vi "Plot Zoom Key Down Detect.vi"(8 "error in (no error)":errorcluster, 10 "Refs":T12, 11 "Loop data in":T1={"TitleCollapse"=refnum, "MouseDownState"=enum."Idle", "RightClickCache"={"Mod"={"Ctrl"=FALSE, "Shift"=FALSE}, "CoordsStart"={"Horizontal"=0, "Vertical"=0}, "CoordsEnd"={"Horizontal"=0, "Vertical"=0}, "PlotAreaBounds"={"Left"=10, "Top"=10, "Right"=0, "Bottom"=0}, "slice"=[]}, "ZoomCache"={"SuppressedPlots"=[], "LeftAxis"={"NeedsRevert?"=FALSE, "Scale Fit"=0, "Range"={"Minimum"=0.0, "Maximum"=0.0, "Increment"=0.0, "Minor Increment"=0.0, "Start"=0.0}}, "RightAxis"={"NeedsRevert?"=FALSE, "Scale Fit"=0, "Range"={"Minimum"=0.0, "Maximum"=0.0, "Increment"=0.0, "Minor Increment"=0.0, "Start"=0.0}}, "Mod"={"Shift"=FALSE}}, "UpdateTime"=0.0, "keyboard"=refnum, "visible?"=FALSE}) -> (0 "error out":errorcluster, 3 "Loop data out":T1={"TitleCollapse"=refnum, "MouseDownState"=enum."Idle", "RightClickCache"={"Mod"={"Ctrl"=FALSE, "Shift"=FALSE}, "CoordsStart"={"Horizontal"=0, "Vertical"=0}, "CoordsEnd"={"Horizontal"=0, "Vertical"=0}, "PlotAreaBounds"={"Left"=10, "Top"=10, "Right"=0, "Bottom"=0}, "slice"=[]}, "ZoomCache"={"SuppressedPlots"=[], "LeftAxis"={"NeedsRevert?"=FALSE, "Scale Fit"=0, "Range"={"Minimum"=0.0, "Maximum"=0.0, "Increment"=0.0, "Minor Increment"=0.0, "Start"=0.0}}, "RightAxis"={"NeedsRevert?"=FALSE, "Scale Fit"=0, "Range"={"Minimum"=0.0, "Maximum"=0.0, "Increment"=0.0, "Minor Increment"=0.0, "Start"=0.0}}, "Mod"={"Shift"=FALSE}}, "UpdateTime"=0.0, "keyboard"=refnum, "visible?"=FALSE})   [LabVIEW 2021, in "RocketPlot.lvlib"]
uses:
  RocketPlot.lvlib
  TypeDefs/Plot UI references.ctl
  Classes/RocketPlotHandle/RocketPlotHandle.lvclass
  <userlib>/bjustice/TipStripOOPanel/Classes/TipPanelHandle/TipPanelHandle.lvclass
  TypeDefs/Plot top row.ctl
  TypeDefs/plot while loop data.ctl
  CollapsePanel/CollapsePanel.lvclass
  TypeDefs/MouseDownState.ctl
  TypeDefs/RightClickCache.ctl
  TypeDefs/RightClickCache PlatMod.ctl
  <vilib>/Utility/miscctls.llb/LVPoint32TypeDef.ctl
  <vilib>/Utility/miscctls.llb/LVRectTypeDef.ctl
  TypeDefs/Slice average.ctl
  TypeDefs/ZoomCache.ctl
  TypeDefs/RangeCache.ctl
  <vilib>/Utility/miscctls.llb/LVRangeTypeDef.ctl
  TypeDefs/ZoomCache PlatMod.ctl
  PlatMods to Zoom mods.vi
  <vilib>/Utility/inputDevices.llb/keyboardAcquire.vi
  Zoom Cache end.vi
  Zoom Cache start.vi
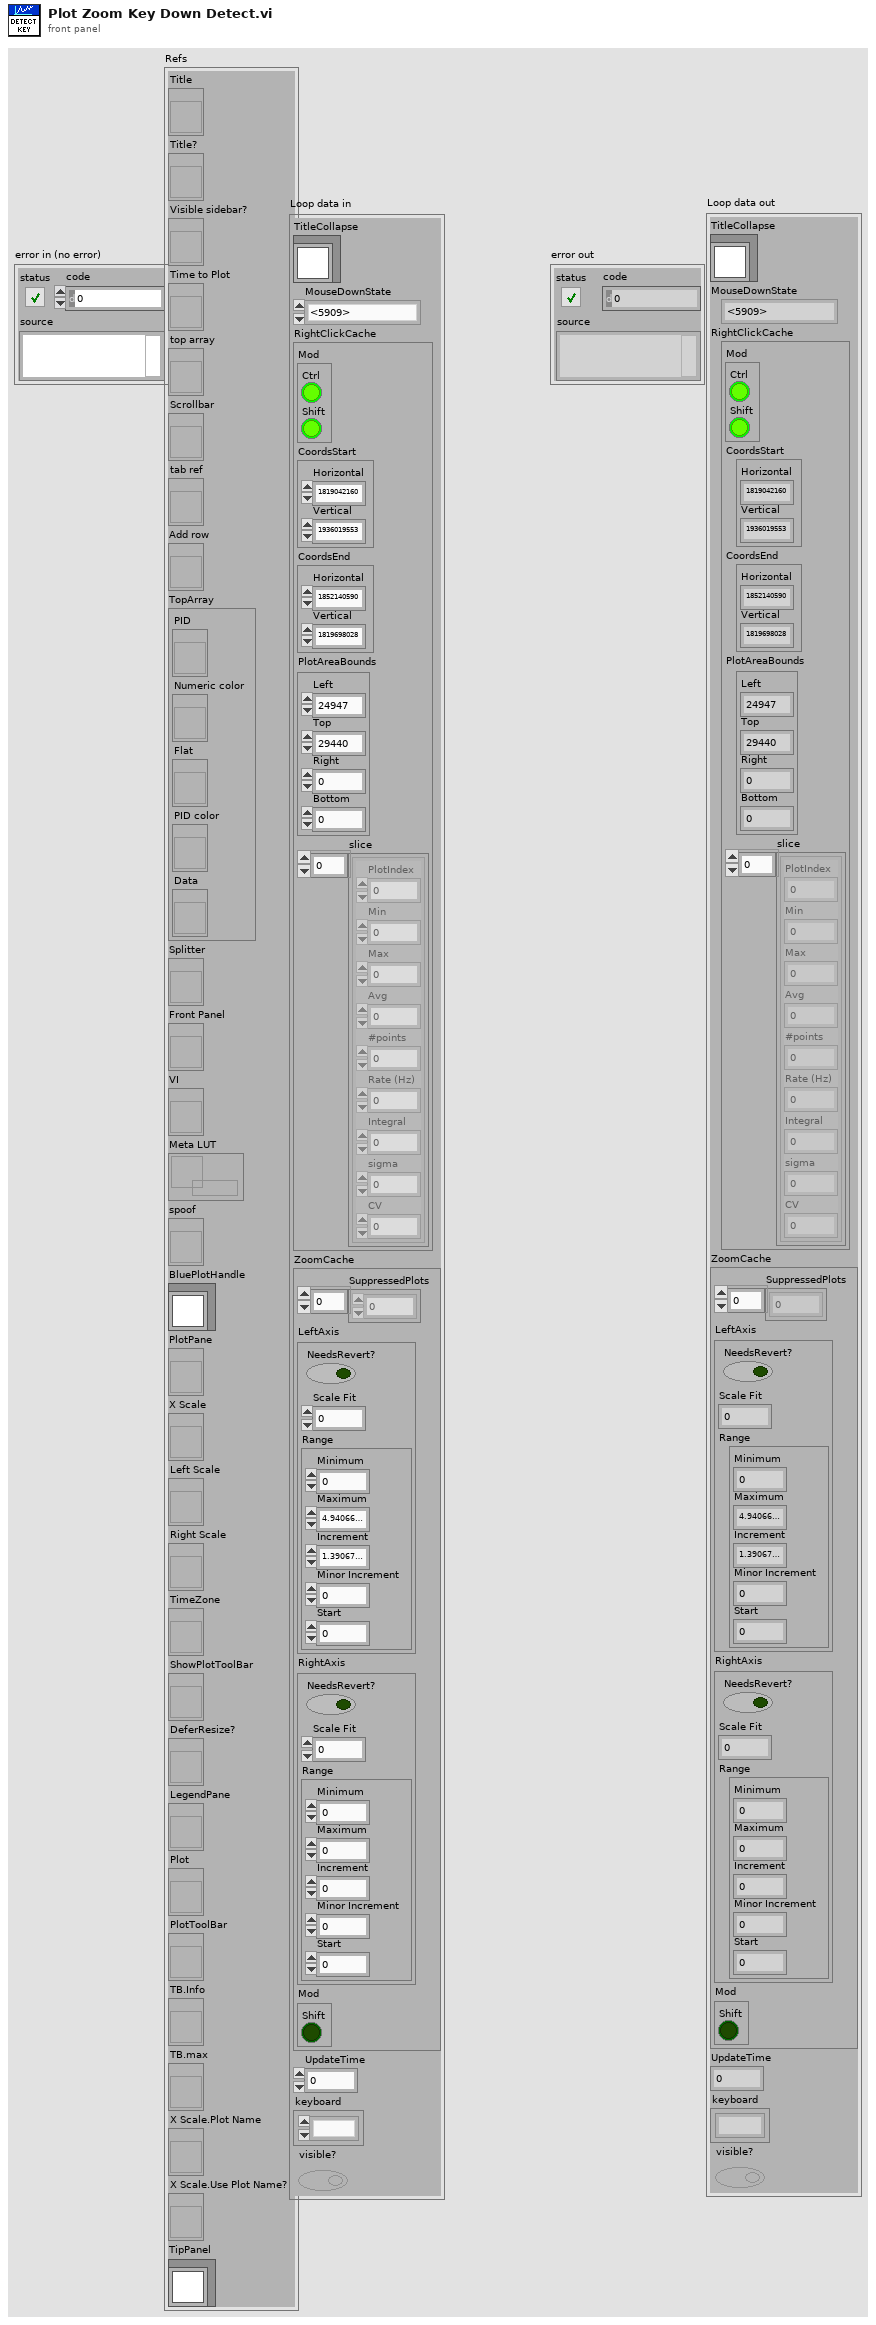
[diagram p1: front panel]
types:
  T1 = typedef "RocketPlot.lvlib/plot while loop data.ctl" = cluster{"TitleCollapse":refnum<class "CollapsePanel.lvclass">, "MouseDownState":T2, "RightClickCache":T3, "ZoomCache":T8, "UpdateTime":dbl, "keyboard":refnum<k1>, "visible?":bool}
  T2 = typedef "RocketPlot.lvlib/MouseDownState.ctl" = enum16{"Idle", "Pan", "Zoom", "Zoom-Post", "RightClick"}
  T3 = typedef "RocketPlot.lvlib/RightClickCache.ctl" = cluster{"Mod":T4, "CoordsStart":T5, "CoordsEnd":T5, "PlotAreaBounds":T6, "slice":T7[]}
  T4 = typedef "RocketPlot.lvlib/RightClickCache PlatMod.ctl" = cluster{"Ctrl":bool, "Shift":bool}
  T5 = typedef "LVPoint32TypeDef.ctl" = cluster{"Horizontal":i32, "Vertical":i32}
  T6 = typedef "LVRectTypeDef.ctl" = cluster{"Left":i16, "Top":i16, "Right":i16, "Bottom":i16}
  T7 = typedef "RocketPlot.lvlib/Slice average.ctl" = cluster{"PlotIndex":i32, "Min":dbl, "Max":dbl, "Avg":dbl, "#points":u32, "Rate (Hz)":dbl, "Integral":dbl, "sigma":dbl, "CV":dbl}
  T8 = typedef "RocketPlot.lvlib/ZoomCache.ctl" = cluster{"SuppressedPlots":i32[], "LeftAxis":T9, "RightAxis":T9, "Mod":T11}
  T9 = typedef "RocketPlot.lvlib/RangeCache.ctl" = cluster{"NeedsRevert?":bool, "Scale Fit":u8, "Range":T10}
  T10 = typedef "LVRangeTypeDef.ctl" = cluster{"Minimum":dbl, "Maximum":dbl, "Increment":dbl, "Minor Increment":dbl, "Start":dbl}
  T11 = typedef "RocketPlot.lvlib/ZoomCache PlatMod.ctl" = cluster{"Shift":bool}
  T12 = typedef "RocketPlot.lvlib/Plot UI references.ctl" = cluster{"Title":refnum<vi>, "Title?":refnum<vi>, "Visible sidebar?":refnum<vi>, "Time to Plot":refnum<vi>, "top array":refnum<vi>, "Scrollbar":refnum<vi>, "tab ref":refnum<vi>, "Add row":refnum<vi>, "TopArray":cluster{"PID":refnum<vi>, "Numeric color":refnum<vi>, "Flat":refnum<vi>, "PID color":refnum<vi>, "Data":refnum<vi>}, "Splitter":refnum<vi>, "Front Panel":refnum<vi>, "VI":refnum<vi>, "Meta LUT":refnum<data-value>, "spoof":refnum<vi>, "BluePlotHandle":refnum<class "RocketPlotHandle.lvclass">, "PlotPane":refnum<vi>, "X Scale":refnum<vi>, "Left Scale":refnum<vi>, "Right Scale":refnum<vi>, "TimeZone":refnum<vi>, "ShowPlotToolBar":refnum<vi>, "DeferResize?":refnum<vi>, "LegendPane":refnum<vi>, "Plot":refnum<vi>, "PlotToolBar":refnum<vi>, "TB.Info":refnum<vi>, "TB.max":refnum<vi>, "X Scale.Plot Name":refnum<vi>, "X Scale.Use Plot Name?":refnum<vi>, "TipPanel":refnum<class "TipPanelHandle.lvclass">}
  T13 = cluster{"Shift":bool, "Ctrl":bool, "Alt":bool, "Cmd":bool, "Opt":bool}
  T14 = enum16{"0", "1", "2", "3", "4", "5", "6", "7", "8", "9", "A", "B", "C", "D", "E", "F", "G", "H", "I", "J", "K", "L", "M", "N", "O", "P", "Q", "R", "S", "T", "U", "V", "W", "X", "Y", "Z", "F1", "F2", "F3", "F4", "F5", "F6", "F7", "F8", "F9", "F10", "F11", "F12", "F13", "F14", "F15", "ADD", "BACK", "BACKSLASH", "CAPITAL", "COMMA", "DECIMAL", "DELETE", "DIVIDE", "DOWN", "END", "EQUALS", "ESCAPE", "GRAVE (`)", "HOME", "INSERT", "LBRACKET", "LCONTROL", "LEFT", "L ALT", "LSHIFT", "LWIN", "MINUS", "MULTIPLY", "NEXT", "NUMLOCK", "NUMPAD_0", "NUMPAD_1", "NUMPAD_2", "NUMPAD_3", "NUMPAD_4", "NUMPAD_5", "NUMPAD_6", "NUMPAD_7", "NUMPAD_8", "NUMPAD_9", "PAUSE", "PERIOD", "PRIOR (PG UP)", "RBRACKET", "RCONTROL", "RETURN", "RIGHT", "R ALT", "RSHIFT", "RWIN", "SCROLL", "SEMICOLON", "SLASH", "SPACE", "SUBTRACT", "TAB", "UP", "ENTER (num pad)", "' (quote)"}
  T15 = enum16{"0", "1", "2", "3", "4", "5", "6", "7", "8", "9", "A", "B", "C", "D", "E", "F", "G", "H", "I", "J", "K", "L", "M", "N", "O", "P", "Q", "R", "S", "T", "U", "V", "W", "X", "Y", "Z", "F1", "F2", "F3", "F4", "F5", "F6", "F7", "F8", "F9", "F10", "F11", "F12", "F13", "F14", "F15", "ADD", "BACK", "BACKSLASH", "CAPITAL", "COMMA", "DECIMAL", "DELETE", "DIVIDE", "DOWN", "END", "EQUALS", "ESCAPE", "GRAVE (`)", "HOME", "INSERT", "LBRACKET", "LCONTROL", "LEFT", "L ALT", "LSHIFT", "LWIN", "MINUS", "MULTIPLY", "NEXT", "NUMLOCK", "NUMPAD_0", "NUMPAD_1", "NUMPAD_2", "NUMPAD_3", "NUMPAD_4", "NUMPAD_5", "NUMPAD_6", "NUMPAD_7", "NUMPAD_8", "NUMPAD_9", "PAUSE", "PERIOD", "PRIOR (PG UP)", "RBRACKET", "RCONTROL", "RETURN", "RIGHT", "R ALT", "RSHIFT", "RWIN", "SCROLL", "SEMICOLON", "SLASH", "SPACE", "SUBTRACT", "TAB", "UP", "ENTER (num pad)", "' (quote)"}[]
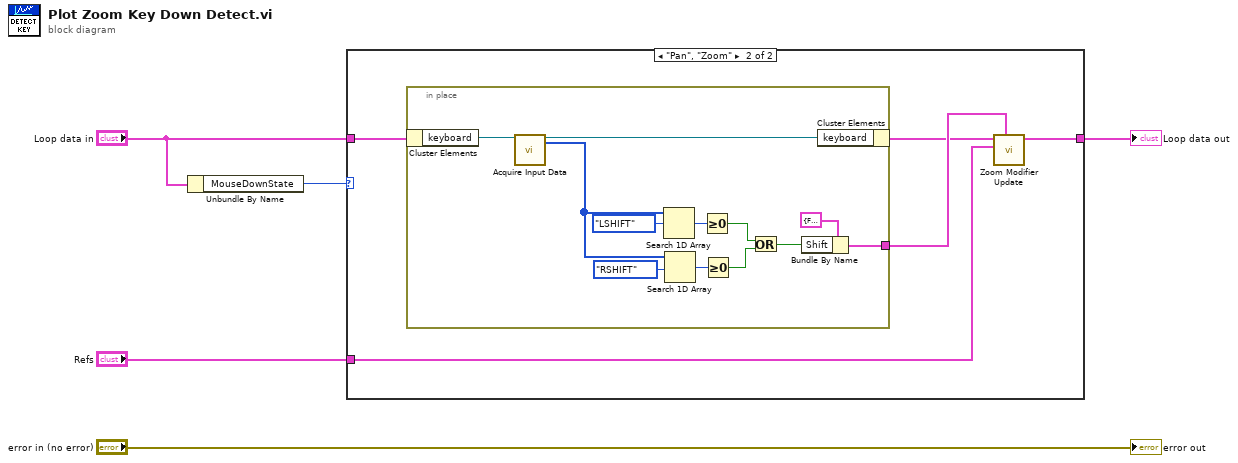
[diagram p0: block diagram]
diagram:
  n1 = Unbundle By Name("Loop data in") -> ("MouseDownState"=w1:T2)
  n2 = case shown="\"Pan\", \"Zoom\"" w1 {
    tunnel: [w6 w9] -> w4
    tunnel: "Refs" -> [_ w11]
    tunnel: "Loop data in" -> [w6 w8]
    frame Default {
    }
    frame "Pan", "Zoom" {
      n3 = in-place {
        in-place-border: [w14] -> w10
        n4 = in-place-cluster #1(w8) -> ("keyboard"=w13:refnum<k1>)
        n5 = call-poly <vilib>:"Acquire Input Data.vi"("device ID"=w13) -> ("device ID"=w12:refnum<k1>, "keys pressed"=w22:T15)  [unwired: 16 in, 1 out]
        n6 = Search 1D Array(1D array=w22, element=T14."LSHIFT") -> (index of element=w21:i32)  [unwired: 1 in]
        n7 = Search 1D Array(1D array=w22, element=T14."RSHIFT") -> (index of element=w20:i32)  [unwired: 1 in]
        n8 = Greater Or Equal To 0?(x=w21) -> (x >= 0?=w19:bool)
        n9 = Greater Or Equal To 0?(x=w20) -> (x >= 0?=w18:bool)
        n10 = Or(x=w19, y=w18) -> (x .or. y?=w16:bool)
        n11 = Bundle By Name(cluster=T13 {"Shift"=FALSE, "Ctrl"=FALSE, "Alt"=FALSE, "Cmd"=FALSE, "Opt"=FALSE} ("PlatMods"), "Shift"=w16) -> (w14:T13)
        n12 = in-place-cluster #1("keyboard"=w12) -> (w7:T1)
      }
      n13 = call "Zoom Modifier Update.vi"("PlatMods"=w10, "Refs"=w11, "Loop data in"=w7) -> ("Loop data out"=w9:T1)  [unwired: 7 in, 1 out]
    }
  }
  "Loop data out" <- w4
  "error out" <- "error in (no error)"
